vi "ShiftRegister.vi"() -> ()   [LabVIEW 2020]
panel:
  out "output cluster":cluster{"led":bool, "termo":dbl}
  out "Array":bool[](array[boolean])
  out "Boolean":bool
  out "concatenated string":string
  out "x+y":i32
  in  "stop":bool
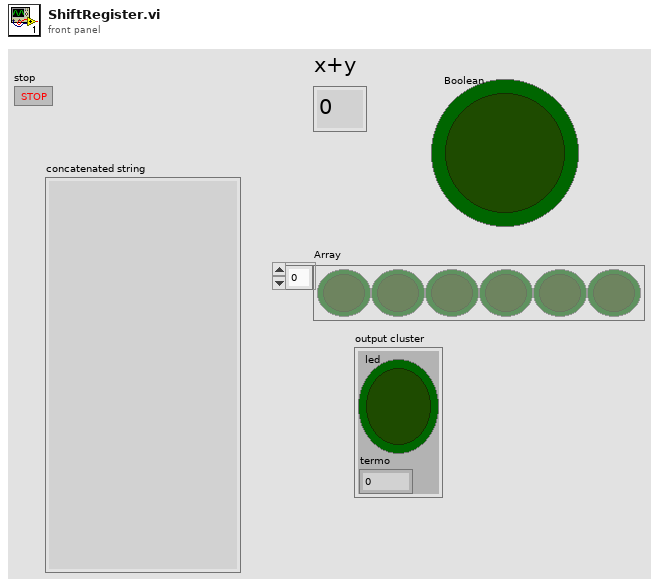
[diagram p1: front panel]
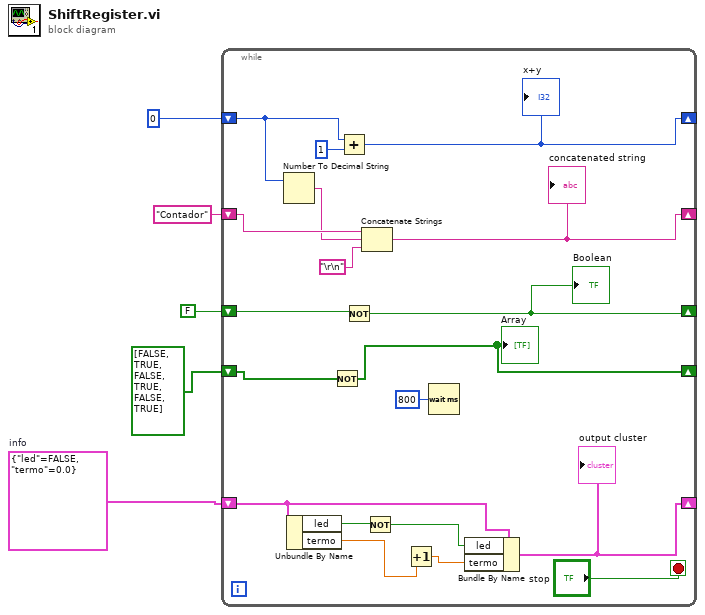
[diagram p0: block diagram]
diagram:
  w1 = cluster{"led":bool, "termo":dbl} {"led"=FALSE, "termo"=0.0}  # info
  n1 = while {
    shift-right: [w22] -> _
    shift-left: 0 -> [w20]
    shift-right: [w16] -> _
    shift-left: "Contador" -> [w19]
    shift-right: [w14] -> _
    shift-left: FALSE -> [w15]
    shift-right: [w12] -> _
    shift-left: bool[] [FALSE, TRUE, FALSE, TRUE, FALSE, TRUE] -> [w13]
    shift-right: [w6] -> _
    shift-left: w1 -> [w9]
    stop <- "stop" stop-if-true
    n2 = Number To Decimal String(number=w20) -> (decimal integer string=w18:string)  [unwired: 1 in]
    n3 = Unbundle By Name(w9) -> ("led"=w11:bool, "termo"=w10:dbl)
    n4 = Not(x=w13) -> (.not. x?=w12:bool[])
    "Array" <- w12
    n5 = Add(x=w20, y=1) -> (x+y=w22:i32)
    "x+y" <- w22
    n6 = Not(x=w15) -> (.not. x?=w14:bool)
    "Boolean" <- w14
    n7 = Concatenate Strings(w19, w18, "\r\n") -> (w16:string)
    "concatenated string" <- w16
    n8 = Not(x=w11) -> (.not. x?=w8:bool)
    n9 = Increment(x=w10) -> (x+1=w7:dbl)
    n10 = Wait (ms)(milliseconds to wait=u32 800) -> ()  [unwired: 1 out]
    n11 = Bundle By Name(cluster=w9, "led"=w8, "termo"=w7) -> (w6:cluster{"led":bool, "termo":dbl})
    "output cluster" <- w6
  }
